vi "Start SLSC Session Daemon.vi"(8 "error in (no error)":errorcluster, 11 "device":refnum<k21>) -> (0 "error out":errorcluster)   [LabVIEW 2015, in "SLSC Switch.lvlib" / "SLSC Session.lvclass"]
uses:
  SLSC Session/SLSC Session.lvclass
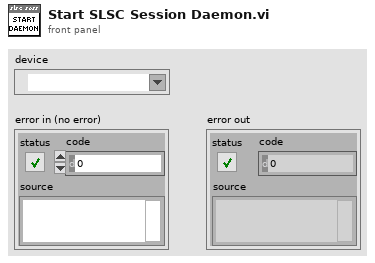
[diagram p1: front panel]
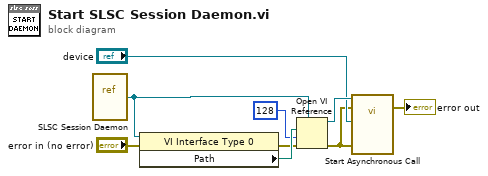
[diagram p0: block diagram]
diagram:
  n1 = vi-ref "SLSC Session Daemon.vi"() -> (w8:refnum<vi>)
  n2 = property class="VI Interface Type 0"(reference=w8, error in="error in (no error)") -> (error out=w6:errorcluster, "Path"=w9:path)  [unwired: 1 out]
  n3 = Open VI Reference(type specifier VI Refnum (for type only)=w8, vi path=w9, options=128, error in (no error)=w6) -> (vi reference=w7:refnum<vi>, error out=w2:errorcluster)  [unwired: 2 in]
  n4 = call-by-ref "Start Asynchronous Call"(reference=w7, error in=w2, 8:"error in (no error)"=w2, "device"="device") -> (error out=→"error out":errorcluster)  [unwired: 9 in, 2 out]
